vi "MidbrainArbiter.vi"(0 "ForebrainInput":dbl[](array[numeric]), 5 "ObstacleAvoid":dbl[](array[numeric]), 7 "S-Wall Follow":dbl[](array[numeric]), 9 "Lane Follow":dbl[](array[numeric]), 11 "Wall Avoid":dbl[](array[numeric]), 12 "P-Wall Follow":dbl[](array[numeric])) -> (8 "Act Command":cluster{"Velocity":dbl, "Direction":dbl})   [LabVIEW 2012]
doc: "This VI arbitrates the one command input form the Forebrain, and a set of inputs from the Limbic and Cerrebellum THINK processes and conducts a voting poll arbitor with input from each to determine the one output command.\n\nInputs: 90 cell arrays of weighted direction commands \n\nOutput: Cluster of desried velocity and direction"
panel:
  out "BrainWave Waveform Graph":dbl[][](graph)
  # "This subVI takes the three\nACT commands; one from the forebrain \nand three from the Midbrain and\naverages them"
  # "Steering angle in\nlocal referance  frame\nwith array slot 45 being\nstraight ahead off bow.\nzero would be 45 deg \nto port, 90 would be 45\nto starboard."
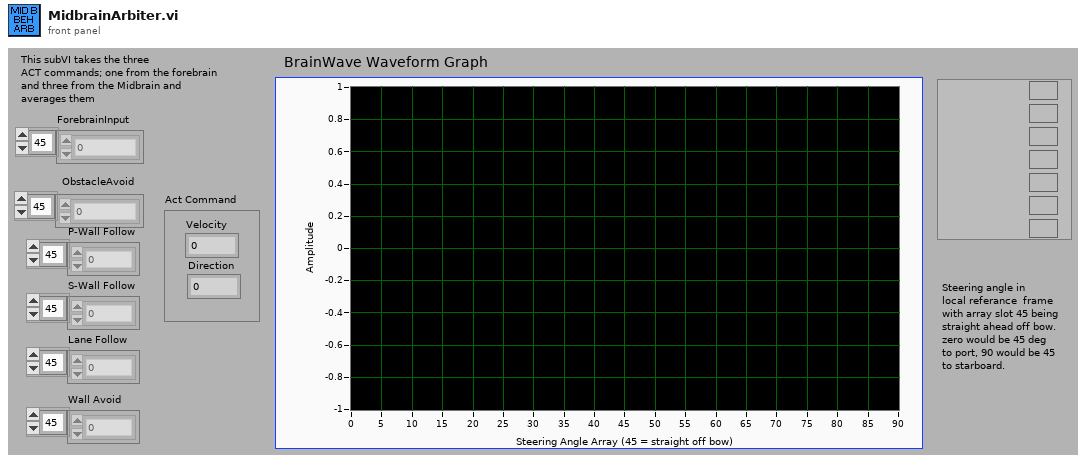
[diagram p1: front panel]
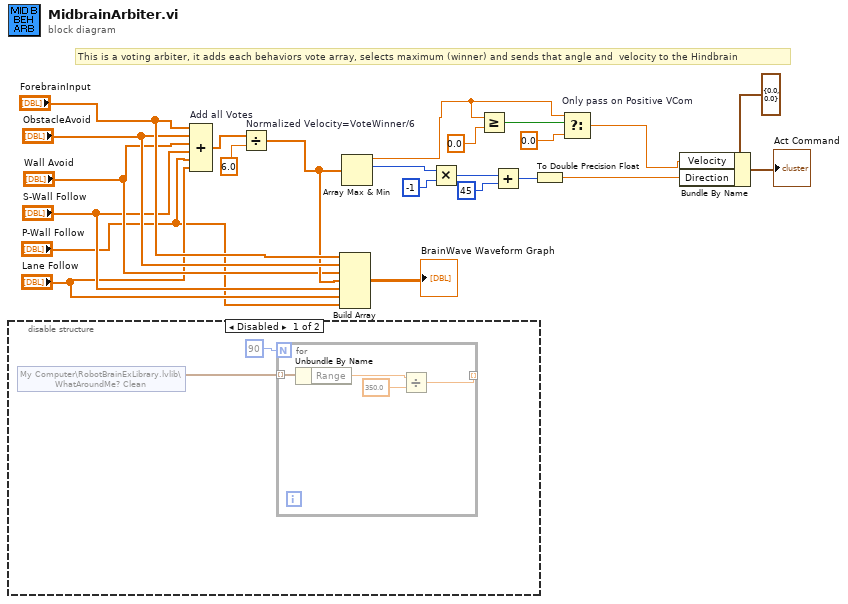
[diagram p0: block diagram]
diagram:
  # "This is a voting arbiter, it adds each behaviors vote array, selects maximum (winner) and sends that angle and  velocity to the Hindbrain"
  n1 = disable-structure shown="Disabled" {
    frame Disabled {
      n2 = shared-variable "My Computer\\RobotBrainExLibrary.lvlib\\WhatAroundMe? Clean"() -> (w24:cluster{"T":dbl, "Range":dbl, "Bearing":dbl}[])  [unwired: 1 in, 1 out]
      n3 = for {
        N: 90 -> [_]
        tunnel: w24 -> [w29] mode=indexing
        tunnel: [w27] -> _ mode=indexing
        n4 = Unbundle By Name(w29) -> ("Range"=w28:dbl)
        n5 = Divide(x=w28, y=350.0) -> (x/y=w27:dbl)
      }
    }
    frame Enabled {
    }
  }
  n6 = Compound Arithmetic op=ADD "Add all Votes"("ForebrainInput", "ObstacleAvoid", "Wall Avoid", "S-Wall Follow", "P-Wall Follow", "Lane Follow") -> (w12:dbl[])
  n7 = Divide "Normalized Velocity=VoteWinner/6"(x=w12, y=6.0) -> (x/y=w5:dbl[])
  n8 = Build Array "Build Array"("ForebrainInput", "ObstacleAvoid", "Wall Avoid", w5, "S-Wall Follow", "Lane Follow", "P-Wall Follow") -> (→"BrainWave Waveform Graph":dbl[][])
  n9 = Array Max & Min(array=w5) -> (max value=w8:dbl, max index (indices)=w21:i32)  [unwired: 2 out]
  n10 = Multiply(x=w21, y=-1) -> (x*y=w19:i32)
  n11 = Greater Or Equal?(x=w8, y=0.0) -> (x >= y?=w9:bool)
  n12 = Add(x=w19, y=45) -> (x+y=w17:i32)
  n13 = To Double Precision Float(number=w17) -> (double precision float=w16:dbl)
  n14 = Select "Only pass on Positive VCom"(t=w8, s=w9, f=0.0) -> (s? t:f=w6:dbl)
  n15 = Bundle By Name(cluster=cluster{"Velocity":dbl, "Direction":dbl} {"Velocity"=0.0, "Direction"=0.0} ("Act Command"), "Velocity"=w6, "Direction"=w16) -> (→"Act Command":cluster{"Velocity":dbl, "Direction":dbl})
